vi "OracleLoop.vi"(8 "Error In":errorcluster, 11 "Message Queues":T1) -> (0 "Error Out":errorcluster)   [LabVIEW 2017, in "Server.lvlib" / "Oracle.lvlib"]
doc: "This Loop is responsible for polling the Oracle Database for new SRs. It will then transfer these SRs to the MHL for further processing.\nThis Loop does not have its own queue. Thats why it is stopped with the \"Stop?\" Global Variable!"
uses:
  Oracle.lvlib
  Message Queue/CommReferences.ctl
  Message Queue/MessageCluster.ctl
  OracleLoopData.ctl
  <vilib>/addons/database/Connection.llb/Conn ObjectReference.ctl
  OracleData.ctl
  TypeDefs/ServerINI.ctl
  <vilib>/Utility/error.llb/Error Cluster From Error Code.vi
  Message Queue/EnqueueMessage(Single).vi
  <vilib>/ErrorRing/Error Ring.xnode
  Message Queue/Message Queue.lvlib
  ErrorLogger/ErrorLogger.lvlib
  <vilib>/addons/database/NI_Database_API.lvlib
  Server.lvlib
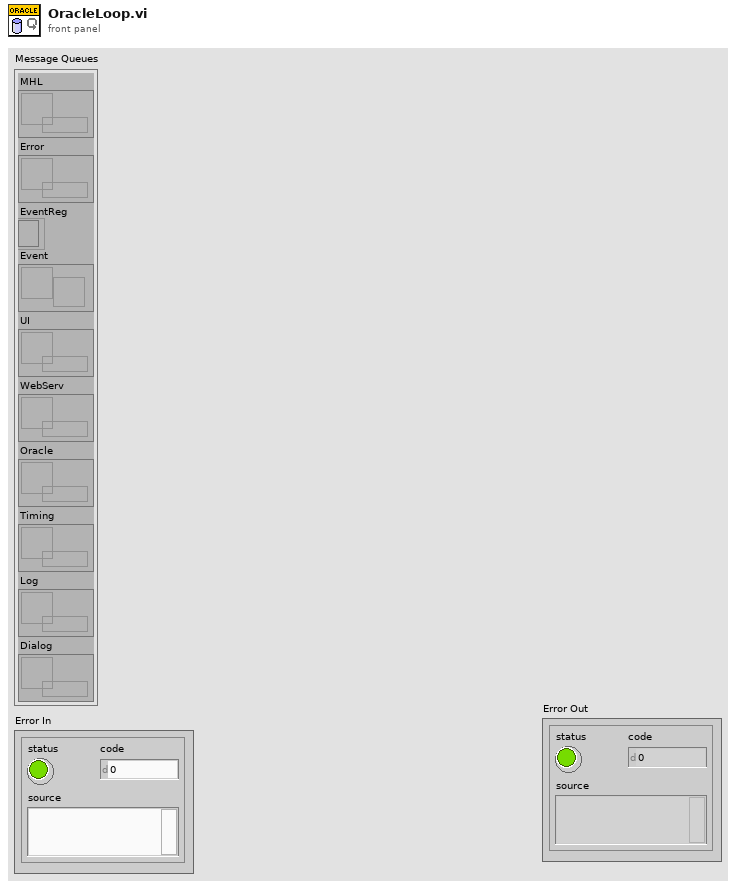
[diagram p1: front panel]
types:
  T1 = typedef "Server.lvlib/Message Queue.lvlib/CommReferences.ctl" = cluster{"MHL":refnum<queue>, "Error":refnum<queue>, "EventReg":refnum<event-registration>, "Event":refnum<user-event>, "UI":refnum<queue>, "WebServ":refnum<queue>, "Oracle":refnum<queue>, "Timing":refnum<queue>, "Log":refnum<queue>, "Dialog":refnum<queue>}
  T2 = typedef "Server.lvlib/Oracle.lvlib/OracleLoopData.ctl" = cluster{"reference":T3, "OracleData":T4}
  T3 = typedef "NI_Database_API.lvlib/Conn ObjectReference.ctl" = refnum<k1>
  T4 = typedef "Server.lvlib/Oracle.lvlib/OracleData.ctl" = cluster{"DBname":string, "User":string, "Password":string}
  T5 = typedef "Server.lvlib/ServerINI.ctl" = cluster{"ClientTimeout (s)":u32, "LogPath":path, "CriticalErrors":i32[], "OracleData":T4}
  T6 = typedef "Server.lvlib/SR List.ctl" = T7[]
  T7 = typedef "Server.lvlib/SR Data.ctl" = cluster{"SR#":dbl, "Group":string, "Owner":string, "Problem Summary":string, "Last Updated":timestamp, "Customer First Name":string, "Customer Last Name":string, "Company":string, "Created On":timestamp, "SR Type":string, "Status":string, "Service Level":string, "Channel":string, "Days Open":dbl}
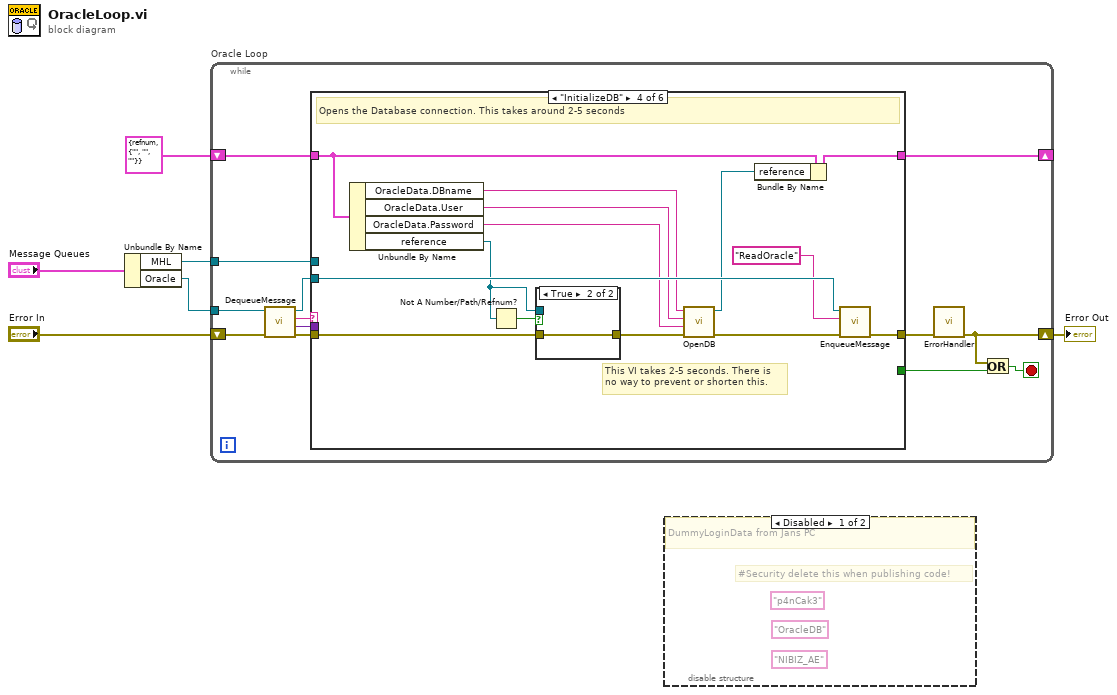
[diagram p0: block diagram]
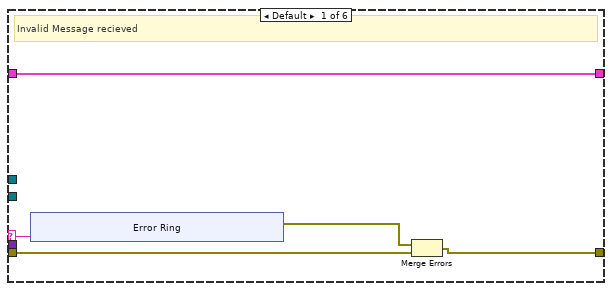
[diagram p3: hidden frame]
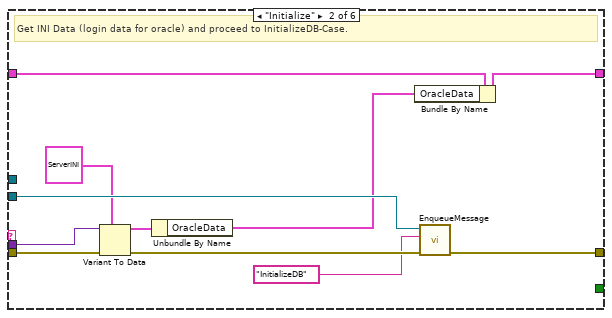
[diagram p4: hidden frame]
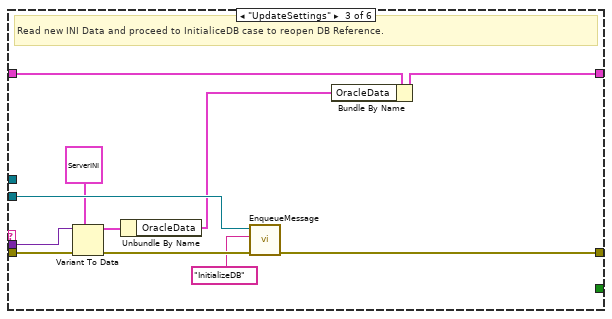
[diagram p5: hidden frame]
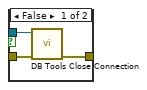
[diagram p6: hidden frame]
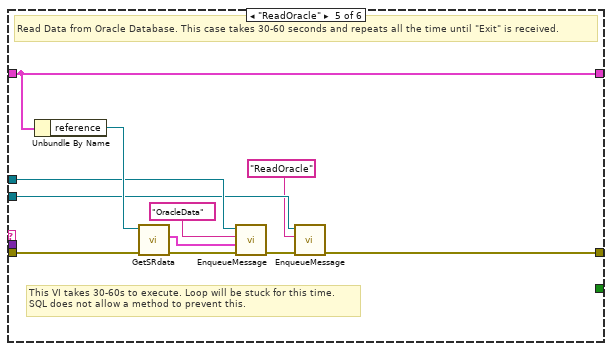
[diagram p7: hidden frame]
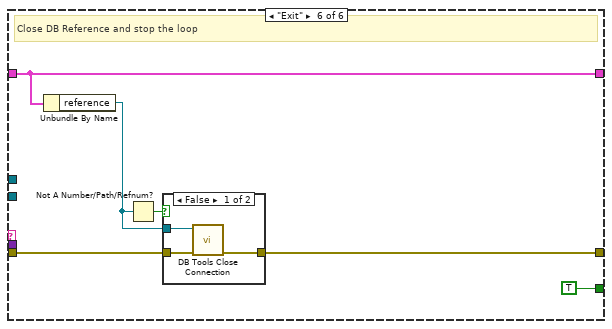
[diagram p8: hidden frame]
diagram:
  n1 = Unbundle By Name("Message Queues") -> ("MHL"=w4:refnum<queue>, "Oracle"=w2:refnum<queue>)
  n2 = while "Oracle Loop" {
    shift-right: [w7] -> w6
    shift-left: "Error In" -> [w19]
    tunnel: w4 -> [w13]
    tunnel: w2 -> [w17]
    shift-right: [w10] -> _
    shift-left: T2 {"reference"=refnum, "OracleData"={"DBname"="", "User"="", "Password"=""}} ("OracleLoopData") -> [w11]
    stop <- w8 stop-if-true
    n3 = call "DequeueMessage.vi"("error in (no error)"=w19, "Message Queue"=w17) -> ("error out"=w18:errorcluster, "Message Data"=w15:variant, "Message"=w16:string, "dup Message Queue"=w9:refnum<queue>)  [unwired: 5 in, 1 out]
    n4 = case shown="\"InitializeDB\"" w16 {
      selector: w16 -> [w23 _ _ _ _ _]
      tunnel: w18 -> [w24 w42 w44 w62 w80 w87]
      tunnel: [w22 w41 w53 w65 w74 w86] -> w12
      tunnel: w15 -> [_ w37 w50 _ _ _]
      tunnel: [_ _ _ _ _ TRUE] -> w14
      tunnel: w13 -> [_ _ _ _ w76 _]
      tunnel: w9 -> [_ w40 w52 w64 w73 _]
      tunnel: [w20 w33 w43 w67 w82 w85] -> w10
      tunnel: w11 -> [w20 w39 w46 w66 w82 w85]
      frame Default {
        # "Invalid Message recieved"
        n5 = xnode "Error Ring"("parameter 0"=w23) -> ("error out"=w21:errorcluster)
        n6 = Merge Errors(w21, w24) -> (w22:errorcluster)
      }
      frame "Initialize" {
        # "Get INI Data (login data for oracle) and proceed to InitializeDB-Case."
        n7 = Variant To Data(error in=w42, type=T5 {"ClientTimeout (s)"=30, "LogPath"=path "C:/Users/jgoebel/Documents/GitHub/AEDashboard/ServerLib/Data/ServerLog.tdms", "CriticalErrors"=[], "OracleData"={"DBname"="", "User"="", "Password"=""}} ("ServerINI"), Variant=w37) -> (data=w35:T5, error out=w38:errorcluster)
        n8 = Unbundle By Name(w35) -> ("OracleData"=w34:T4)
        n9 = Bundle By Name(cluster=w39, "OracleData"=w34) -> (w33:T2)
        n10 = call-poly "EnqueueMessage.vi"("error in (no error)"=w38, "Message"="InitializeDB", "Message Queue"=w40) -> ("error out"=w41:errorcluster)  [unwired: 7 in, 1 out]
      }
      frame "UpdateSettings" {
        # "Read new INI Data and proceed to InitialiceDB case to reopen DB Reference."
        n11 = Variant To Data(error in=w44, type=T5 {"ClientTimeout (s)"=30, "LogPath"=path "C:/Users/jgoebel/Documents/GitHub/AEDashboard/ServerLib/Data/ServerLog.tdms", "CriticalErrors"=[], "OracleData"={"DBname"="", "User"="", "Password"=""}} ("ServerINI"), Variant=w50) -> (data=w48:T5, error out=w51:errorcluster)
        n12 = Unbundle By Name(w48) -> ("OracleData"=w47:T4)
        n13 = call-poly "EnqueueMessage.vi"("error in (no error)"=w51, "Message"="InitializeDB", "Message Queue"=w52) -> ("error out"=w53:errorcluster)  [unwired: 7 in, 1 out]
        n14 = Bundle By Name(cluster=w46, "OracleData"=w47) -> (w43:T2)
      }
      frame "InitializeDB" {
        # "This VI takes 2-5 seconds. There is \nno way to prevent or shorten this."
        # "Opens the Database connection. This takes around 2-5 seconds"
        n15 = Unbundle By Name(w66) -> ("OracleData.DBname"=w60:string, "OracleData.User"=w59:string, "OracleData.Password"=w58:string, "reference"=w55:T3)
        n16 = Not A Number/Path/Refnum?(number/path/refnum=w55) -> (NaN/Path/Refnum?=w54:bool)
        n17 = case shown="True" w54 {
          tunnel: w62 -> [w70 w71]
          tunnel: [w69 w71] -> w56
          tunnel: w55 -> [w68 _]
          frame False {
            n18 = call <vilib>:"DB Tools Close Connection.vi"("error in (no error)"=w70, "connection reference"=w68) -> ("error out"=w69:errorcluster)  [unwired: 5 in]
          }
          frame True {
          }
        }
        n19 = call "OpenDB.vi"("Error In"=w56, "Password"=w58, "Username"=w59, "DB-Name"=w60) -> ("error out"=w61:errorcluster, "connection reference"=w57:T3)  [unwired: 6 in]
        n20 = Bundle By Name(cluster=w66, "reference"=w57) -> (w67:T2)
        n21 = call-poly "EnqueueMessage.vi"("error in (no error)"=w61, "Message"="ReadOracle", "Message Queue"=w64) -> ("error out"=w65:errorcluster)  [unwired: 7 in, 1 out]
      }
      frame "ReadOracle" {
        # "This VI takes 30-60s to execute. Loop will be stuck for this time.\nSQL does not allow a method to prevent this."
        # "Read Data from Oracle Database. This case takes 30-60 seconds and repeats all the time until \"Exit\" is received."
        n22 = Unbundle By Name(w82) -> ("reference"=w78:T3)
        n23 = call "GetSRdata.vi"("Error In"=w80, "reference"=w78) -> ("Error Out"=w79:errorcluster, "SRList"=w77:T6)  [unwired: 8 in]
        n24 = call-poly "EnqueueMessage.vi"("error in (no error)"=w79, "Message Data"=w77, "Message"="OracleData", "Message Queue"=w76) -> ("error out"=w75:errorcluster)  [unwired: 6 in, 1 out]
        n25 = call-poly "EnqueueMessage.vi"("error in (no error)"=w75, "Message"="ReadOracle", "Message Queue"=w73) -> ("error out"=w74:errorcluster)  [unwired: 7 in, 1 out]
      }
      frame "Exit" {
        # "Close DB Reference and stop the loop"
        n26 = Unbundle By Name(w85) -> ("reference"=w83:T3)
        n27 = Not A Number/Path/Refnum?(number/path/refnum=w83) -> (NaN/Path/Refnum?=w84:bool)
        n28 = case shown="False" w84 {
          tunnel: w87 -> [w91 w92]
          tunnel: [w90 w92] -> w86
          tunnel: w83 -> [w89 _]
          frame False {
            n29 = call <vilib>:"DB Tools Close Connection.vi"("error in (no error)"=w91, "connection reference"=w89) -> ("error out"=w90:errorcluster)  [unwired: 5 in]
          }
          frame True {
          }
        }
      }
    }
    n30 = call "ErrorHandler.vi"("error in (no error)"=w12) -> ("error out"=w7:errorcluster)  [unwired: 10 in]
    n31 = Or(x=w7, y=w14) -> (x .or. y?=w8:bool)
  }
  "Error Out" <- w6
  n32 = disable-structure shown="Disabled" {
    frame Disabled {
      (unwired) "NIBIZ_AE" ("Username")
      (unwired) "OracleDB" ("DB-Name")
      (unwired) "p4nCak3" ("Password")
      # "#Security delete this when publishing code!"
      # "DummyLoginData from Jans PC"
    }
    frame Enabled {
    }
  }
